vi "example (stacked and flat structures).vi"() -> ()   [LabVIEW 2021]
panel:
  out "Tank 2":dbl(slide) scale=0.0..10.0
  in  "stop 2":bool
  out "Boolean 2":bool
  out "Knob 2":dbl(knob) scale=0.0..10.0
  in  "stop":bool
  out "Tank":dbl(slide) scale=0.0..10.0
  out "Boolean":bool
  out "Knob":dbl(knob) scale=0.0..10.0
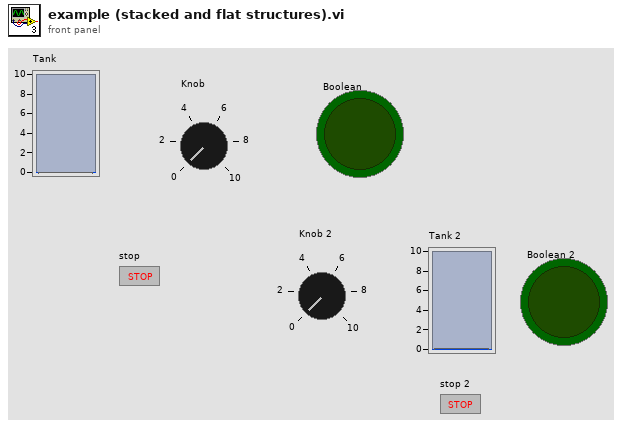
[diagram p1: front panel]
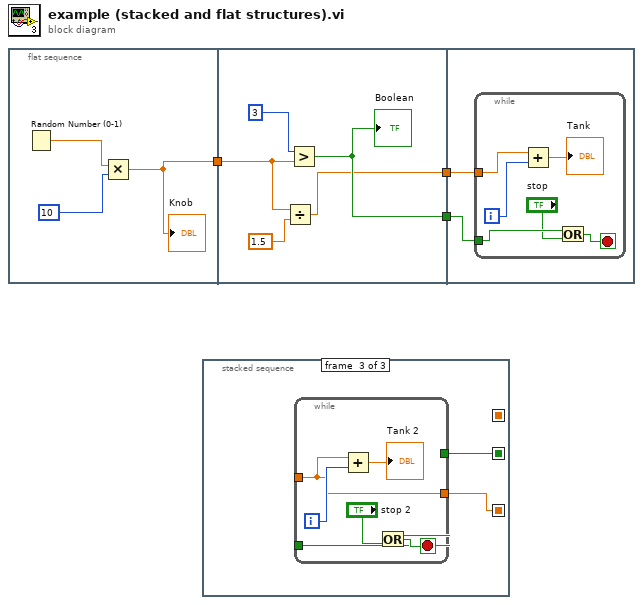
[diagram p0: block diagram]
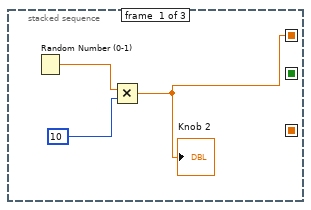
[diagram p2: hidden frame]
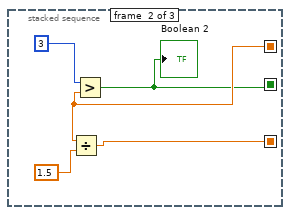
[diagram p3: hidden frame]
diagram:
  n1 = flat-sequence {
    tunnel: [w4] -> w3
    tunnel: w3 -> [w9]
    tunnel: [w10] -> w2
    tunnel: [w7] -> w1
    tunnel: w2 -> [w13]
    tunnel: w1 -> [w12]
    frame #0 {
      n2 = Random Number (0-1)() -> (number: 0 to 1=w6:dbl)
      n3 = Multiply(x=w6, y=10) -> (x*y=w4:dbl)
      "Knob" <- w4
    }
    frame #1 {
      n4 = Divide(x=w9, y=1.5) -> (x/y=w7:dbl)
      n5 = Greater?(x=3, y=w9) -> (0:w10:bool)
      "Boolean" <- w10
    }
    frame #2 {
      n6 = while {
        tunnel: w13 -> [w15]
        tunnel: w12 -> [w17]
        i -> [w18]
        stop <- w16 stop-if-true
        n7 = Add(x=w17, y=w18) -> (x+y=→"Tank":dbl)
        n8 = Or(x=w15, y="stop") -> (x .or. y?=w16:bool)
      }
    }
  }
  n9 = stacked-sequence {
    seq-local: [w20 _ _] -> [_ w25 _]
    seq-local: [_ w24 _] -> [_ _ w29]
    seq-local: [_ w23 _] -> [_ _ w28]
    frame #0 {
      n10 = Random Number (0-1)() -> (number: 0 to 1=w22:dbl)
      n11 = Multiply(x=w22, y=10) -> (x*y=w20:dbl)
      "Knob 2" <- w20
    }
    frame #1 {
      n12 = Divide(x=w25, y=1.5) -> (x/y=w23:dbl)
      n13 = Greater?(x=3, y=w25) -> (0:w24:bool)
      "Boolean 2" <- w24
    }
    frame #2 {
      n14 = while {
        tunnel: [w31] -> _
        tunnel: [w30] -> _
        tunnel: w29 -> [w31]
        tunnel: w28 -> [w30]
        i -> [w34]
        stop <- w33 stop-if-true
        n15 = Add(x=w30, y=w34) -> (x+y=→"Tank 2":dbl)
        n16 = Or(x=w31, y="stop 2") -> (x .or. y?=w33:bool)
      }
    }
  }
